vi "Get Yaw.vi"() -> (0 "Angle":dbl)   [LabVIEW 2016]
uses:
  <vilib>/Rock Robotics/Network Tables/SD Write Number.vi
  navX-MXP Library/navX-MXP IMU.lvlib
panel:
  in  "Gyro Offset":dbl
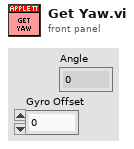
[diagram p1: front panel]
types:
  T1 = typedef "navX-MXP IMU.lvlib/navX Serial DevRef.ctl" = cluster{"SerialPortRef":T2, "Board Information":T3, "Status":T4, "Offsets":cluster{"Yaw":dbl, "Quat W":dbl, "Quat X":dbl, "Quat Y":dbl, "Quat Z":dbl}, "Update Rate (4Hz-60Hz)":u8, "Nav6Mode (YPR)":T8, "refnum name":string, "error":errorcluster}
  T2 = typedef "WPI_SerialPortRef.ctl" = cluster{"DevStatus":errorcluster, "Serial Port Name":refnum<visa-resource-name>}
  T3 = typedef "navX-MXP IMU.lvlib/navX Board Information.ctl" = cluster{"WhoAmI (50 | 0x32)":u8, "Board Revision":u8, "Firmware Major Version":u8, "Firmware Minor Version":u8}
  T4 = typedef "navX-MXP IMU.lvlib/navX Status Data.ctl" = cluster{"Update Rate Hz":u8, "Accelerometer Full-Scale Range":u8, "Gyro Full-Scale Range":u16, "NAVX_OP_STATUS":T5, "NAVX_CAL_STATUS":T6, "NAVX_SELFTEST_STATUS":u8, "NAVX_SENSOR_STATUS":T7}
  T5 = typedef "navX-MXP IMU.lvlib/navX NAVX_OP_STATUS.ctl" = u8
  T6 = typedef "navX-MXP IMU.lvlib/navX NAVX_CAL_STATUS.ctl" = u8
  T7 = typedef "navX-MXP IMU.lvlib/navX NAVX_SENSOR_STATUS.ctl" = cluster{"MOVING":bool, "YAW_STABLE":bool, "MAG_DISTURBANCE":bool, "ALTITUDE_VALID":bool, "SEALEVEL_PRESS_SET":bool, "FUSED_HEADING_VALID":bool}
  T8 = typedef "navX-MXP IMU.lvlib/navX Serial Mode.ctl" = enum16{"YPR", "Gyro", "Quaternion"}
  T9 = typedef "navX-MXP IMU.lvlib/navX YPRH Data.ctl" = cluster{"Yaw":dbl, "Pitch":dbl, "Roll":dbl, "Heading":dbl}
  T10 = typedef "navX-MXP IMU.lvlib/navX SPI DevRef.ctl" = cluster{"SPIDevRef":T11, "Board Information":T3, "Status":T4, "Offsets":cluster{"Yaw":dbl, "Quat W":dbl, "Quat X":dbl, "Quat Y":dbl, "Quat Z":dbl}, "Update Rate (4Hz-60Hz)":u8, "refnum name":string, "error":errorcluster}
  T11 = typedef "WPI_SPIDevRef.ctl" = cluster{"DevStatus":errorcluster, "Handle":i32, "SPI Bus":T12}
  T12 = typedef "spi_bus.ctl" = enum16{"SPI On-Board, CS0", "SPI On-Board, CS1", "SPI On-Board, CS2", "SPI On-Board, CS3", "SPI MXP", "Invalid"}
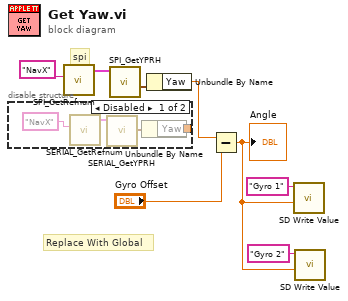
[diagram p0: block diagram]
diagram:
  # "Replace With Global"
  # "spi"
  n1 = disable-structure shown="Disabled" {
    disable-tunnel: [w12 _] -> _
    frame Disabled {
      n2 = call "SERIAL_GetRefnum.vi"("refnum name"="NavX") -> ("navX DevRef"=w9:T1)  [unwired: 9 in, 1 out]
      n3 = call "SERIAL_GetYPRH.vi"("navX Ref Object"=w9) -> ("YPRH"=w10:T9)  [unwired: 9 in, 1 out]
      n4 = Unbundle By Name(w10) -> ("Yaw"=w12:dbl)
    }
    frame Enabled {
    }
  }
  n5 = call "SPI_GetRefnum.vi"("refnum name"="NavX") -> ("navX DevRef"=w6:T10)  [unwired: 9 in, 1 out]
  n6 = call "SPI_GetYPRH.vi"("navX DevRef"=w6) -> ("YPRH"=w7:T9)  [unwired: 8 in, 2 out]
  n7 = Unbundle By Name(w7) -> ("Yaw"=w5:dbl)
  n8 = Subtract(x=w5, y="Gyro Offset") -> (x-y=w4:dbl)
  "Angle" <- w4
  n9 = call-poly <vilib>:"SD Write Value.vi"("Numeric"=w4, "Name"="Gyro 1") -> ()  [unwired: 8 in, 2 out]
  n10 = call-poly <vilib>:"SD Write Value.vi"("Numeric"=w4, "Name"="Gyro 2") -> ()  [unwired: 8 in, 2 out]
